vi "ELVIS III v1.0 Reserve PWM.vi"(7 "Allow multiple opens?":bool, 8 "error in (no error)":errorcluster, 10 "PWM Channel":T2, 11 "myRIO FPGA Ref In":T1) -> (0 "error out":errorcluster)   [LabVIEW 2021]
uses:
  <vilib>/myRIO/Common/Instrument Driver Framework/myRIO v1.0/PWM/typedefs/PWM Channels Enum.ctl
  <vilib>/myRIO/Common/Instrument Driver Framework/Utilities/typedefs/Generic FPGA Reference.ctl
  <vilib>/myRIO/Common/Instrument Driver Framework/ELVIS III v1.0/Resource Manager/vis/ELVIS III v1.0 Create Configuration List.vi
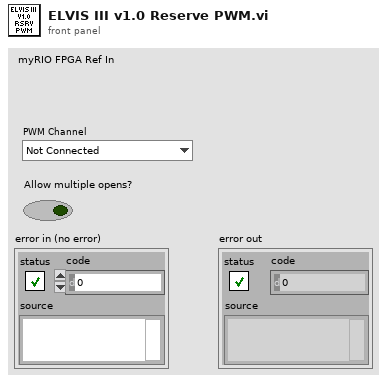
[diagram p1: front panel]
types:
  T1 = typedef "Generic FPGA Reference.ctl" = refnum<k20>
  T2 = typedef "PWM Channels Enum.ctl" = enum16{"Not Connected", "C/PWM0", "C/PWM1", "A/PWM0", "A/PWM1", "A/PWM2", "A/PWM3", "A/PWM4", "A/PWM5", "A/PWM6", "A/PWM7", "A/PWM8", "A/PWM9", "A/PWM10", "A/PWM11", "A/PWM12", "A/PWM13", "A/PWM14", "A/PWM15", "A/PWM16", "A/PWM17", "A/PWM18", "A/PWM19", "B/PWM0", "B/PWM1", "B/PWM2", "B/PWM3", "B/PWM4", "B/PWM5", "B/PWM6", "B/PWM7", "B/PWM8", "B/PWM9", "B/PWM10", "B/PWM11", "B/PWM12", "B/PWM13", "B/PWM14", "B/PWM15", "B/PWM16", "B/PWM17", "B/PWM18", "B/PWM19", "PWM/PWM0", "PWM/PWM1", "PWM/PWM2", "PWM/PWM3", "PWM/PWM4", "PWM/PWM5", "PWM/PWM6", "PWM/PWM7", "PWM/PWM8", "PWM/PWM9"}
  T3 = typedef "ELVIS III v1.0 Channel Reservation List.ctl" = T4[]
  T4 = typedef "ELVIS III v1.0 Channel Reservation Info.ctl" = cluster{"Channel Name":string, "Connector":T5, "MutexIDs":u32[]}
  T5 = typedef "ELVIS III v1.0 Connector List.ctl" = enum32{"None", "ConnectorA", "ConnectorB"}
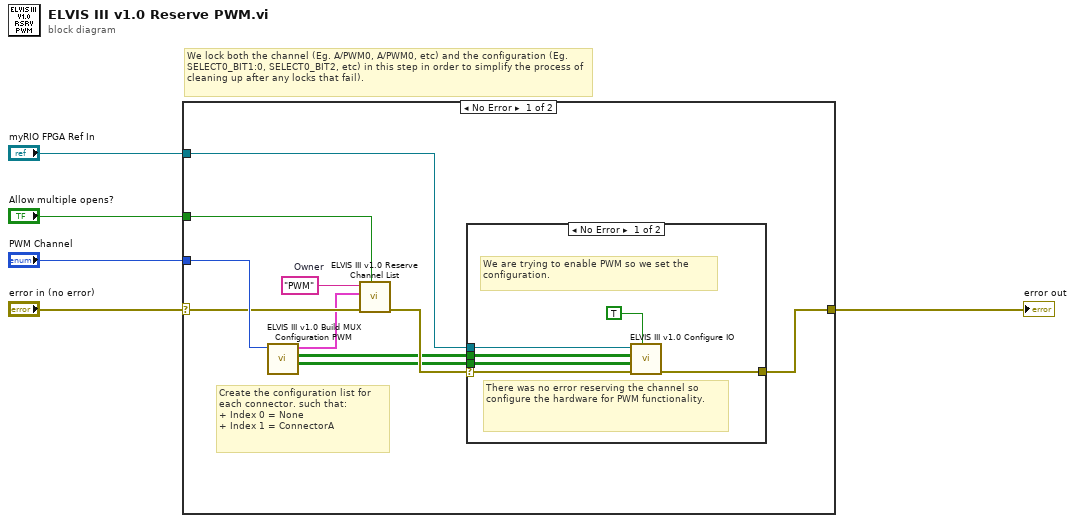
[diagram p0: block diagram]
diagram:
  # "We lock both the channel (Eg. A/PWM0, A/PWM0, etc) and the configuration (Eg. SELECT0_BIT1:0, SELECT0_BIT2, etc) in this step in order to simplify the process of cleaning up after any locks that fail)."
  n1 = case shown="No Error" "error in (no error)" {
    selector: "error in (no error)" -> [w10 w23]
    tunnel: "myRIO FPGA Ref In" -> [w12 _]
    tunnel: "PWM Channel" -> [w15 _]
    tunnel: [w11 w23] -> w3
    tunnel: "Allow multiple opens?" -> [w14 _]
    frame No Error {
      w13 = "PWM"  # Owner
      # "Create the configuration list for each connector. such that:\n+ Index 0 = None\n+ Index 1 = ConnectorA"
      n2 = call <vilib>:"ELVIS III v1.0 Build MUX Configuration PWM.vi"("Channel"=w15) -> ("Configuration Bitmask Array"=w8:bool[][], "Configuration BitCode Array"=w6:bool[][], "Channel Reservation List"=w7:T3)  [unwired: 8 in]
      n3 = call <vilib>:"ELVIS III v1.0 Reserve Channel List.vi"("Allow multiple opens?"=w14, "error in (no error)"=w10, "Channel Reservation List"=w7, "Owner"=w13) -> ("error out"=w9:errorcluster)  [unwired: 7 in]
      n4 = case shown="No Error" w9 {
        selector: w9 -> [w18 w22]
        tunnel: w12 -> [w20 _]
        tunnel: [w19 w22] -> w11
        tunnel: w6 -> [w17 _]
        tunnel: w8 -> [w16 _]
        frame No Error {
          # "There was no error reserving the channel so configure the hardware for PWM functionality."
          # "We are trying to enable PWM so we set the configuration."
          n5 = call <vilib>:"ELVIS III v1.0 Configure IO.vi"("Value"=TRUE ("Clear?"), "error in (no error)"=w18, "Bitmask Array"=w16, "Bitcode Array"=w17, "myRIO FPGA Ref In"=w20) -> ("error out"=w19:errorcluster)  [unwired: 6 in]
        }
        frame Error {
        }
      }
    }
    frame Error {
      # "Nothing to do since there is an incoming error."
    }
  }
  "error out" <- w3
